vi "numCmd_Recv_OneDbl.vi"(7 "Command Name":string, 11 "Initial Value":dbl) -> (0 "error out":errorcluster, 2 "Changed":bool, 3 "Value":dbl)   [LabVIEW 2019, in "Trajectory_Library.lvlib"]
uses:
  Trajectory_Library.lvlib
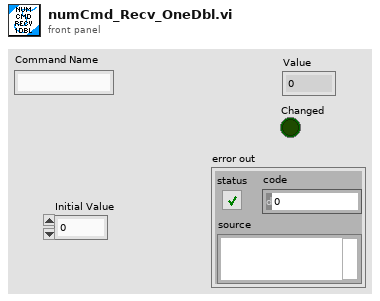
[diagram p1: front panel]
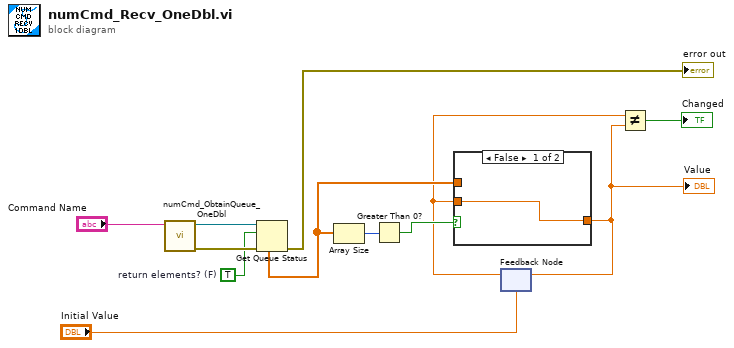
[diagram p0: block diagram]
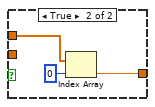
[diagram p2: hidden frame]
diagram:
  w6 = TRUE  # return elements? (F)
  n1 = call "numCmd_ObtainQueue_OneDbl.vi"("Command Name"="Command Name") -> ("error out"=w11:errorcluster, "queue out"=w12:refnum<queue>)  [unwired: 9 in]
  n2 = Get Queue Status(queue=w12, return elements? (F)=w6, error in (no error)=w11) -> (error out=→"error out":errorcluster, elements=w8:dbl[])  [unwired: 6 out]
  n3 = Array Size(array=w8) -> (size(s)=w10:i32)
  n4 = Greater Than 0?(x=w10) -> (x > 0?=w9:bool)
  n5 = feedback #1("Initial Value") -> (w7:dbl)
  n6 = case shown="False" w9 {
    tunnel: w8 -> [_ w16]
    tunnel: [w13 w14] -> w2
    tunnel: w7 -> [w13 _]
    frame False {
    }
    frame True {
      n7 = Index Array(array=w16, index=0) -> (element=w14:dbl)
    }
  }
  "Value" <- w2
  n8 = feedback-in #1(w2) -> ()
  n9 = Not Equal?(x=w7, y=w2) -> (x != y?=→"Changed":bool)
